vi "Tree_MoveItem_withChildren.vi"(8 "Error In":errorcluster, 9 "End Index":i32, 10 "Start Index":i32, 11 "Tree Refnum IN":refnum<vi>) -> (0 "Error Out":errorcluster, 2 "Moved Tag":string, 3 "Tree Refnum OUT":refnum<vi>)   [LabVIEW 2012]
doc: "SciScan 1.2 160622\nThis VI Moves the child form the original position (in row number), to the final position (in row number).\nIf the specified row values are out of range, and error is generated"
panel:
  in  "Tree 2":string(tree)
  in  "Tree":string(tree)
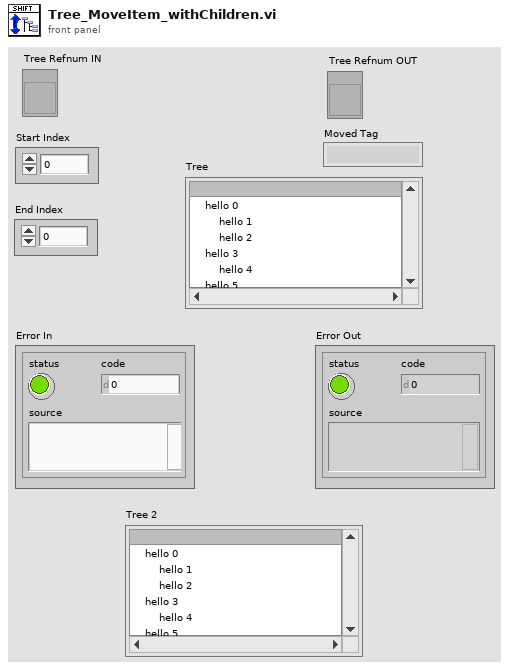
[diagram p1: front panel]
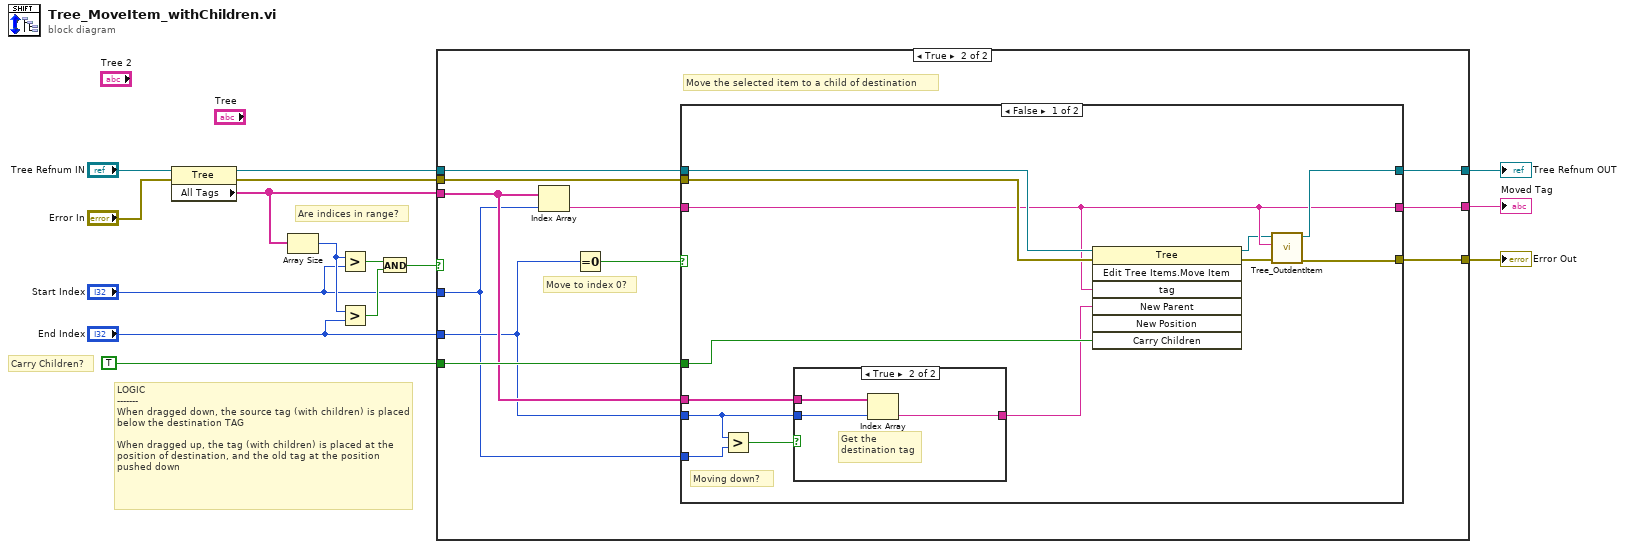
[diagram p0: block diagram]
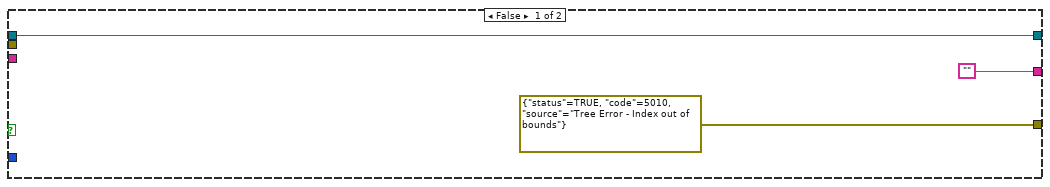
[diagram p2: hidden frame]
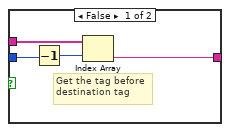
[diagram p3: hidden frame]
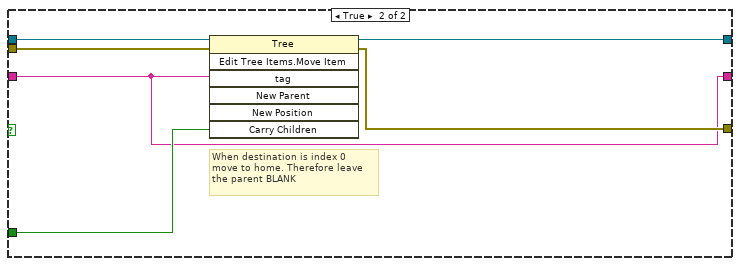
[diagram p4: hidden frame]
diagram:
  # "LOGIC\n-------\nWhen dragged down, the source tag (with children) is placed below the destination TAG\n\nWhen dragged up, the tag (with children) is placed at the position of destination, and the old tag at the position pushed down"
  # "Carry Children?"
  # "Are indices in range?"
  n1 = property class="Tree"(reference="Tree Refnum IN", error in="Error In") -> (reference out=w9:refnum<vi>, error out=w10:errorcluster, "All Tags"=w6:string[])
  n2 = Array Size(array=w6) -> (size(s)=w13:i32)
  n3 = Greater?(x=w13, y="Start Index") -> (0:w14:bool)
  n4 = Greater?(x=w13, y="End Index") -> (0:w12:bool)
  n5 = And(x=w14, y=w12) -> (x .and. y?=w11:bool)
  n6 = case shown="True" w11 {
    tunnel: w10 -> [_ w26]
    tunnel: w9 -> [w18 w27]
    tunnel: "End Index" -> [_ w21]
    tunnel: "Start Index" -> [_ w20]
    tunnel: w6 -> [_ w22]
    tunnel: TRUE ("Carry Children?") -> [_ w25]
    tunnel: [w18 w24] -> w5
    tunnel: [errorcluster {"status"=TRUE, "code"=5010, "source"="Tree Error - Index out of bounds"} ("error out") w23] -> w4
    tunnel: ["" w19] -> w1
    frame False {
    }
    frame True {
      # "Move to index 0?"
      # "Move the selected item to a child of destination"
      n7 = Index Array(array=w22, index=w20) -> (element=w28:string)
      n8 = Equal To 0?(x=w21) -> (x = 0?=w29:bool)
      n9 = case shown="False" w29 {
        tunnel: w28 -> [w31 w50]
        tunnel: w27 -> [w35 w55]
        tunnel: w26 -> [w34 w54]
        tunnel: w25 -> [w42 w53]
        tunnel: [w38 w52] -> w24
        tunnel: [w37 w51] -> w23
        tunnel: w22 -> [w41 _]
        tunnel: w21 -> [w33 _]
        tunnel: w20 -> [w39 _]
        tunnel: [w31 w50] -> w19
        frame False {
          # "Moving down?"
          n10 = Greater?(x=w33, y=w39) -> (0:w40:bool)
          n11 = case shown="True" w40 {
            tunnel: w41 -> [w46 w49]
            tunnel: w33 -> [w45 w47]
            tunnel: [w44 w48] -> w32
            frame False {
              # "Get the tag before\ndestination tag"
              n12 = Decrement(x=w45) -> (x-1=w43:i32)
              n13 = Index Array(array=w46, index=w43) -> (element=w44:string)
            }
            frame True {
              # "Get the \ndestination tag"
              n14 = Index Array(array=w49, index=w47) -> (element=w48:string)
            }
          }
          n15 = invoke class="Tree" method="Edit Tree Items.Move Item"(reference=w35, error in=w34, "tag"=w31, "New Parent"=w32, "Carry Children"=w42) -> (reference out=w30:refnum<vi>, error out=w36:errorcluster)  [unwired: 2 in, 5 out]
          n16 = call "Tree_OutdentItem.vi"("Error In"=w36, "TagToOutdent"=w31, "Tree Refnum"=w30) -> ("Error Out"=w37:errorcluster, "Tree Refnum OUT"=w38:refnum<vi>)  [unwired: 7 in]
        }
        frame True {
          # "When destination is index 0\nmove to home. Therefore leave\nthe parent BLANK"
          n17 = invoke class="Tree" method="Edit Tree Items.Move Item"(reference=w55, error in=w54, "tag"=w50, "Carry Children"=w53) -> (reference out=w52:refnum<vi>, error out=w51:errorcluster)  [unwired: 3 in, 5 out]
        }
      }
    }
  }
  "Tree Refnum OUT" <- w5
  "Error Out" <- w4
  "Moved Tag" <- w1
